vi "Open Motors.vi"() -> (2 "Right":T1={"DeviceStatus"={"status"=FALSE, "code"=0, "source"=""}, "Type"=enum."PWM", "PWM"={"PWM Channel"=enum."Invalid", "DeadBand"={"Name"="", "maxPositivePwm"=0, "minPositivePwm"=0, "centerPwm"=0, "maxNegativePwm"=0, "minNegativePwm"=0, "angularRange"=0}}, "CAN"={"Device Number"=0, "SetOutput VI Ref"=variant(refnum<vi> refnum), "GetOutput VI Ref"=variant(refnum<vi> refnum), "Enable VI Ref"=variant(refnum<vi> refnum), "Disable VI Ref"=variant(refnum<vi> refnum), "Data"=variant}, "Invert"=FALSE, "DIO PWM"={"PWM \"Enable\" Channel"=enum."Invalid", "DIOChannel"=enum."Invalid", "PWM Rate"=0.0}}, 3 "Left":T1={"DeviceStatus"={"status"=FALSE, "code"=0, "source"=""}, "Type"=enum."PWM", "PWM"={"PWM Channel"=enum."Invalid", "DeadBand"={"Name"="", "maxPositivePwm"=0, "minPositivePwm"=0, "centerPwm"=0, "maxNegativePwm"=0, "minNegativePwm"=0, "angularRange"=0}}, "CAN"={"Device Number"=0, "SetOutput VI Ref"=variant(refnum<vi> refnum), "GetOutput VI Ref"=variant(refnum<vi> refnum), "Enable VI Ref"=variant(refnum<vi> refnum), "Disable VI Ref"=variant(refnum<vi> refnum), "Data"=variant}, "Invert"=FALSE, "DIO PWM"={"PWM \"Enable\" Channel"=enum."Invalid", "DIOChannel"=enum."Invalid", "PWM Rate"=0.0}})   [LabVIEW 2019]
uses:
  <vilib>/Rock Robotics/WPI/MotorControl/WPI_MotorControlDeviceRef.ctl
  <vilib>/Rock Robotics/WPI/MotorControl/WPI_MotorControlType.ctl
  <vilib>/Rock Robotics/SystemInterfaces/DIO/FPGA_DIOPWMChannel.ctl
  <vilib>/Rock Robotics/WPI/PWM/WPI_PWMDeadband.ctl
  <vilib>/Rock Robotics/SystemInterfaces/DIO/FPGA_DIOChannel.ctl
  <vilib>/Rock Robotics/WPI/ThirdParty/REV Robotics/SPARK MAX/Typedef/Spark MAX Idle Mode.ctl
  <vilib>/Rock Robotics/WPI/ThirdParty/REV Robotics/SPARK MAX/Typedef/Spark MAX Motor Type.ctl
panel:
  in  "PID Constants":T6={"P Gain"=0.0005, "I Gain"=0.0, "D Gain"=0.0, "F Gain"=0.00017, "I Zone"=0.0, "Min Output"=-1.0, "Max Output"=1.0}
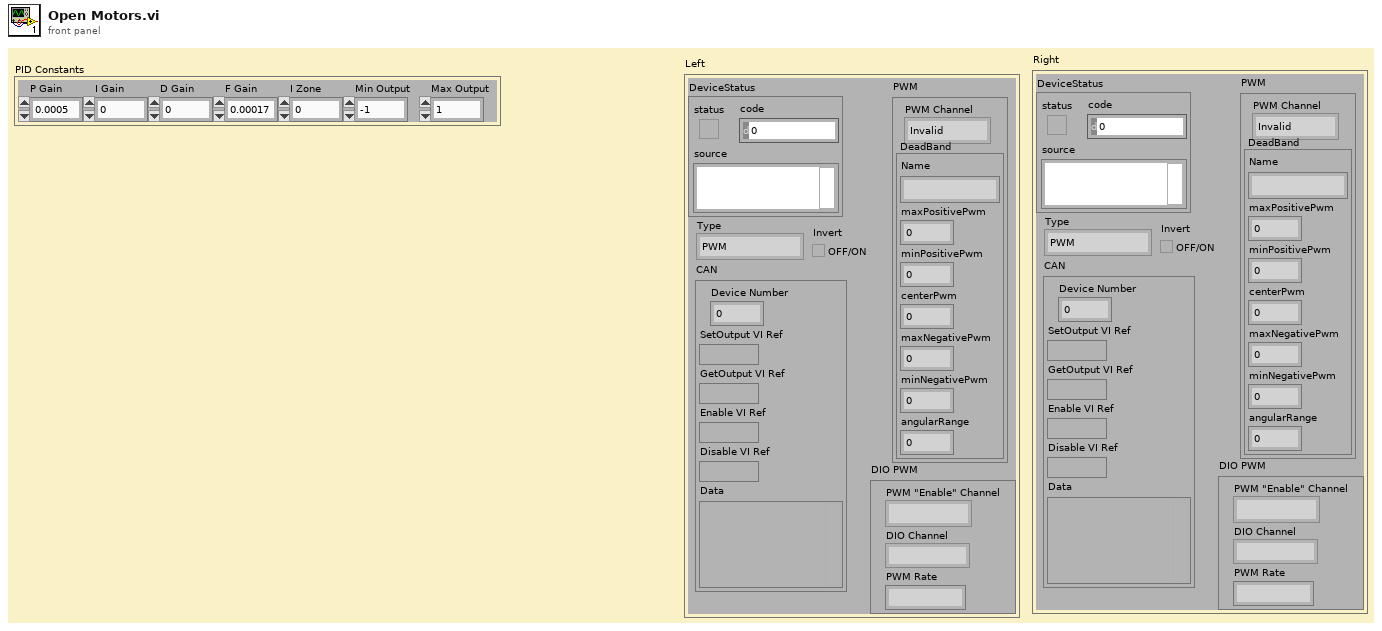
[diagram p1: front panel]
types:
  T1 = typedef "WPI_MotorControlDeviceRef.ctl" = cluster{"DeviceStatus":errorcluster, "Type":T2, "PWM":cluster{"PWM Channel":T3, "DeadBand":T4}, "CAN":cluster{"Device Number":u8, "SetOutput VI Ref":variant, "GetOutput VI Ref":variant, "Enable VI Ref":variant, "Disable VI Ref":variant, "Data":variant}, "Invert":bool, "DIO PWM":cluster{"PWM \"Enable\" Channel":T3, "DIOChannel":T5, "PWM Rate":dbl}}
  T2 = typedef "WPI_MotorControlType.ctl" = enum16{"PWM", "CAN", "DIO PWM"}
  T3 = typedef "FPGA_DIOPWMChannel.ctl" = enum8{"PWM 0", "PWM 1", "PWM 2", "PWM 3", "PWM 4", "PWM 5", "PWM 6", "PWM 7", "PWM 8", "PWM 9", "PWM MXP 0", "PWM MXP 1", "PWM MXP 2", "PWM MXP 3", "PWM MXP 4", "PWM MXP 5", "PWM MXP 6", "PWM MXP 7", "PWM MXP 8", "PWM MXP 9", "Invalid"}
  T4 = typedef "WPI_PWMDeadband.ctl" = cluster{"Name":string, "maxPositivePwm":i32, "minPositivePwm":i32, "centerPwm":i32, "maxNegativePwm":i32, "minNegativePwm":i32, "angularRange":u16}
  T5 = typedef "FPGA_DIOChannel.ctl" = enum8{"DIO 0", "DIO 1", "DIO 2", "DIO 3", "DIO 4", "DIO 5", "DIO 6", "DIO 7", "DIO 8", "DIO 9", "DIO MXP 0", "DIO MXP 1", "DIO MXP 2", "DIO MXP 3", "DIO MXP 4", "DIO MXP 5", "DIO MXP 6", "DIO MXP 7", "DIO MXP 8", "DIO MXP 9", "DIO MXP 10", "DIO MXP 11", "DIO MXP 12", "DIO MXP 13", "DIO MXP 14", "DIO MXP 15", "SPI Port CS1", "SPI Port CS2", "SPI Port CS3", "SPI Port MISO", "SPI Port MOSI", "Invalid"}
  T6 = cluster{"P Gain":dbl, "I Gain":dbl, "D Gain":dbl, "F Gain":dbl, "I Zone":dbl, "Min Output":dbl, "Max Output":dbl}
  T7 = typedef "Spark MAX Motor Type.ctl" = enum16{"Brushed", "Brushless"}
  T8 = typedef "Spark MAX Idle Mode.ctl" = enum16{"Coast", "Brake"}
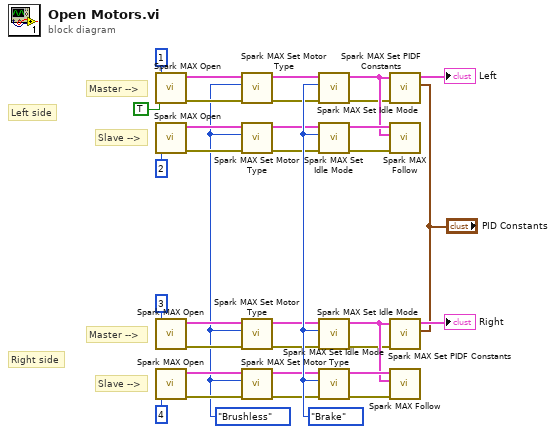
[diagram p0: block diagram]
diagram:
  w1 = Spark_MAX_Motor_Type."Brushless" ("Motor Type")
  w19 = Spark_MAX_Idle_Mode."Brake" ("Coast/Brake")
  # "Slave -->"
  # "Left side"
  # "Master -->"
  # "Slave -->"
  # "Right side"
  # "Master -->"
  n1 = call <vilib>:"Spark MAX Open.vi"("Invert"=TRUE, "Device Number"=u8 1) -> ("error out"=w15:errorcluster, "MotorControlDeviceRef"=w17:T1)  [unwired: 8 in]
  n2 = call <vilib>:"Spark MAX Open.vi"("Device Number"=u8 2) -> ("error out"=w12:errorcluster, "MotorControlDeviceRef"=w13:T1)  [unwired: 9 in]
  n3 = call <vilib>:"Spark MAX Open.vi"("Device Number"=u8 3) -> ("error out"=w8:errorcluster, "MotorControlDeviceRef"=w9:T1)  [unwired: 9 in]
  n4 = call <vilib>:"Spark MAX Open.vi"("Device Number"=u8 4) -> ("error out"=w4:errorcluster, "MotorControlDeviceRef"=w5:T1)  [unwired: 9 in]
  n5 = call <vilib>:"Spark MAX Set Motor Type.vi"("error in (no error)"=w15, "Motor Type"=w1, "MotorControlDevRef"=w17) -> ("error out"=w14:errorcluster, "MotorControlDeviceRef"=w16:T1)  [unwired: 7 in]
  n6 = call <vilib>:"Spark MAX Set Motor Type.vi"("error in (no error)"=w12, "Motor Type"=w1, "MotorControlDevRef"=w13) -> ("error out"=w10:errorcluster, "MotorControlDeviceRef"=w11:T1)  [unwired: 7 in]
  n7 = call <vilib>:"Spark MAX Set Motor Type.vi"("error in (no error)"=w8, "Motor Type"=w1, "MotorControlDevRef"=w9) -> ("error out"=w6:errorcluster, "MotorControlDeviceRef"=w7:T1)  [unwired: 7 in]
  n8 = call <vilib>:"Spark MAX Set Motor Type.vi"("error in (no error)"=w4, "Motor Type"=w1, "MotorControlDevRef"=w5) -> ("error out"=w2:errorcluster, "MotorControlDeviceRef"=w3:T1)  [unwired: 7 in]
  n9 = call <vilib>:"Spark MAX Set Idle Mode.vi"("error in (no error)"=w14, "Idle Mode"=w19, "MotorControlDeviceRef in"=w16) -> ("error out"=w22:errorcluster, "MotorControlDeviceRef out"=w23:T1)  [unwired: 7 in]
  n10 = call <vilib>:"Spark MAX Set Idle Mode.vi"("error in (no error)"=w10, "Idle Mode"=w19, "MotorControlDeviceRef in"=w11) -> ("error out"=w24:errorcluster, "MotorControlDeviceRef out"=w25:T1)  [unwired: 7 in]
  n11 = call <vilib>:"Spark MAX Set Idle Mode.vi"("error in (no error)"=w6, "Idle Mode"=w19, "MotorControlDeviceRef in"=w7) -> ("error out"=w29:errorcluster, "MotorControlDeviceRef out"=w30:T1)  [unwired: 7 in]
  n12 = call <vilib>:"Spark MAX Set Idle Mode.vi"("error in (no error)"=w2, "Idle Mode"=w19, "MotorControlDeviceRef in"=w3) -> ("error out"=w31:errorcluster, "MotorControlDeviceRef out"=w32:T1)  [unwired: 7 in]
  n13 = call <vilib>:"Spark MAX Set PIDF Constants.vi"("error in"=w22, "PID Constants"="PID Constants", "MotorControlDeviceRef"=w23) -> ("MotorControlDeviceRef"=→"Left":T1)  [unwired: 7 in, 1 out]
  n14 = call <vilib>:"Spark MAX Follow.vi"("error in (no error)"=w24, "Master Controller"=w23, "MotorControlDeviceRef"=w25) -> ()  [unwired: 7 in, 2 out]
  n15 = call <vilib>:"Spark MAX Set PIDF Constants.vi"("error in"=w29, "PID Constants"="PID Constants", "MotorControlDeviceRef"=w30) -> ("MotorControlDeviceRef"=→"Right":T1)  [unwired: 7 in, 1 out]
  n16 = call <vilib>:"Spark MAX Follow.vi"("error in (no error)"=w31, "Master Controller"=w30, "MotorControlDeviceRef"=w32) -> ()  [unwired: 7 in, 2 out]
